vi "Write Parameters from Steps.vi"(8 "error in (no error)":errorcluster, 10 "Parameters from Steps":T1[](array[typedef]), 11 "Scan SBlock in":refnum<class "Scan SBlock.lvclass">) -> (0 "error out":errorcluster, 3 "Scan SBlock out":refnum<class "Scan SBlock.lvclass">)   [LabVIEW 2020, in "TALOS.lvlib" / "Run Utilities.lvlib" / "Scan SBlock.lvclass"]
uses:
  Scan SBlock.lvclass
  Advanced Parameters.ctl
  Advanced Panel Parameter Mode.ctl
  Scan SBlock.lvclass/Scan SBlock.ctl
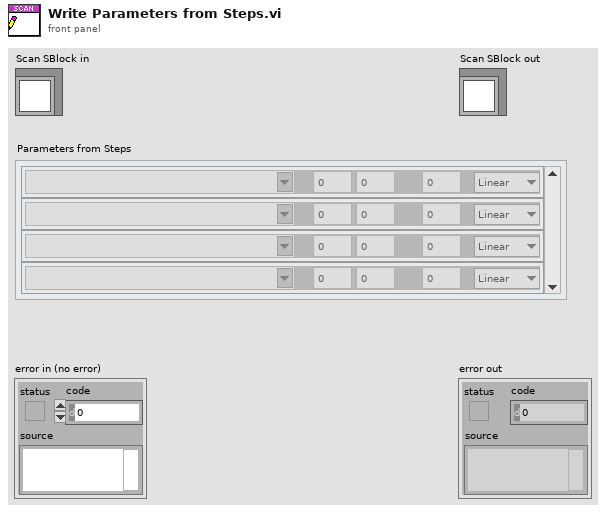
[diagram p1: front panel]
types:
  T1 = typedef "TALOS.lvlib/Run Utilities.lvlib/Scan SBlock.lvclass/Advanced Parameters.ctl" = cluster{"Param":string, "From":dbl, "To":dbl, "Step":dbl, "Mode":T2}
  T2 = typedef "TALOS.lvlib/Run Utilities.lvlib/Scan SBlock.lvclass/Advanced Panel Parameter Mode.ctl" = enum16{"Linear", "Log", "LINKED"}
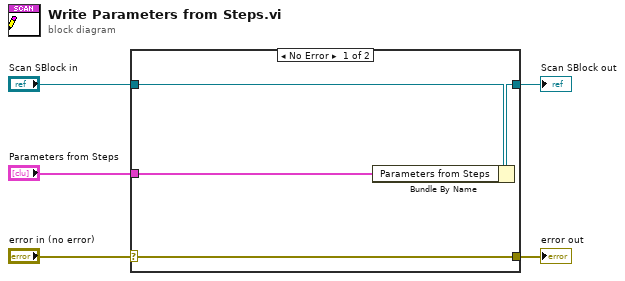
[diagram p0: block diagram]
diagram:
  n1 = case shown="No Error" "error in (no error)" {
    selector: "error in (no error)" -> [w9 w10]
    tunnel: [w9 w10] -> w4
    tunnel: [w7 w11] -> w2
    tunnel: "Scan SBlock in" -> [w8 w11]
    tunnel: "Parameters from Steps" -> [w6 _]
    frame No Error {
      n2 = Bundle By Name(cluster=w8, "Parameters from Steps"=w6) -> (w7:refnum<class "Scan SBlock.lvclass">)
    }
    frame Error {
    }
  }
  "error out" <- w4
  "Scan SBlock out" <- w2
